vi "PKG_IMC_GetADMulParam.vi"(5 "ArrNum":i32, 6 "data":u16[](array[numeric])=[0, 0, 0, 0], 7 "len":u16, 9 "axis":u16, 10 "addr":u16, 11 "Handle":u32) -> (2 "function return":i32, 3 "Handle out":u32)   [LabVIEW 2011, in "IMC_Pkg4xxx.lvlib"]
doc: "PKG_IMC_GetADMulParam(IMC_HANDLE Handle, WR_MUL_DES pdes[], int ArrNum);"
uses:
  IMC_Pkg4xxx.lvlib
  IMC_Pkg4xxx.dll
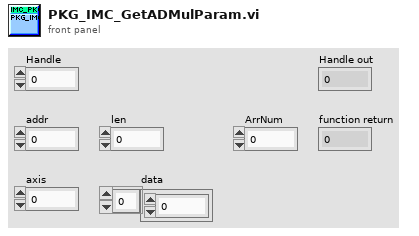
[diagram p1: front panel]
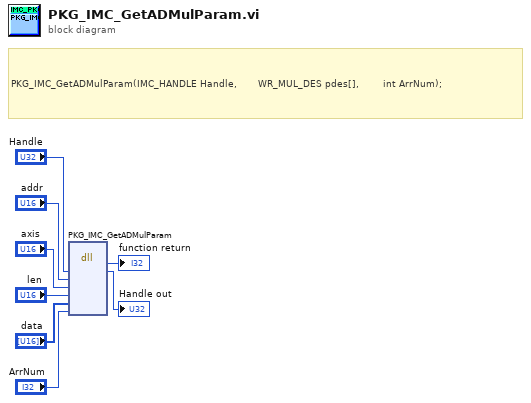
[diagram p0: block diagram]
diagram:
  # "PKG_IMC_GetADMulParam(IMC_HANDLE Handle, \t\t\t\t\t\tWR_MUL_DES pdes[], \t\t\t\t\t\t\tint ArrNum);"
  n1 = dll-call lib="PTH1mabs F光盘刻录\niMC MotionIMCNet_V4.0IMCAppincLabviewIMC_PKG4xxxIMC_PKG4xxx\nIMC_Pkg4xxx.*" fn="PKG_IMC_GetADMulParam"("Handle"="Handle", "addr"="addr", "axis"="axis", "len"="len", "data"="data", "ArrNum"="ArrNum") -> (→"function return":i32, "Handle"=→"Handle out":u32)  [unwired: 8 in, 2 out]
